vi "MultiPotentialStep.vi"() -> ()   [LabVIEW 2023]
uses:
  Sub_Vi/TypeDefs/Display.ctl
  Sub_Vi/TypeDefs/ChangeOnFly.ctl
  Sub_Vi/TypeDefs/Settings.ctl
  Sub_Vi/TypeDefs/WayPointCluster.ctl
  Settings.vi
panel:
  in  "t4 (s)":dbl
  in  "t3 (s)":dbl
  in  "t2 (s)":dbl
  in  "t1 (s)":dbl
  in  "E4 (V)":dbl
  in  "E2 (V)":dbl
  in  "E3 (V)":dbl
  in  "E1 (V)":dbl
  in  "SaveData?":bool=TRUE
  in  "WayPointCluster":T1
  in  "SettingsCluster":T2={"Sample Rate (us)"=1, "Samples Per Data Point (int, power of 2)"=1000, "DistanceToBulk (um)"=-1.0, "HoldTimeScaler"=1, "SaveData"=TRUE, "DistanceToBulk (um) 2"=-1.0, "DistanceToBulk (um) 3"=-1.0}
  in  "ChangeonFly":T3
  in  "Display Cluster":T4
  in  "stop":bool
  in  "Tab Control":enum32{"Current Followers", "Piezos"}(tab)
  out "E-t":dbl[](graph)
  out "i-t":dbl[](graph)
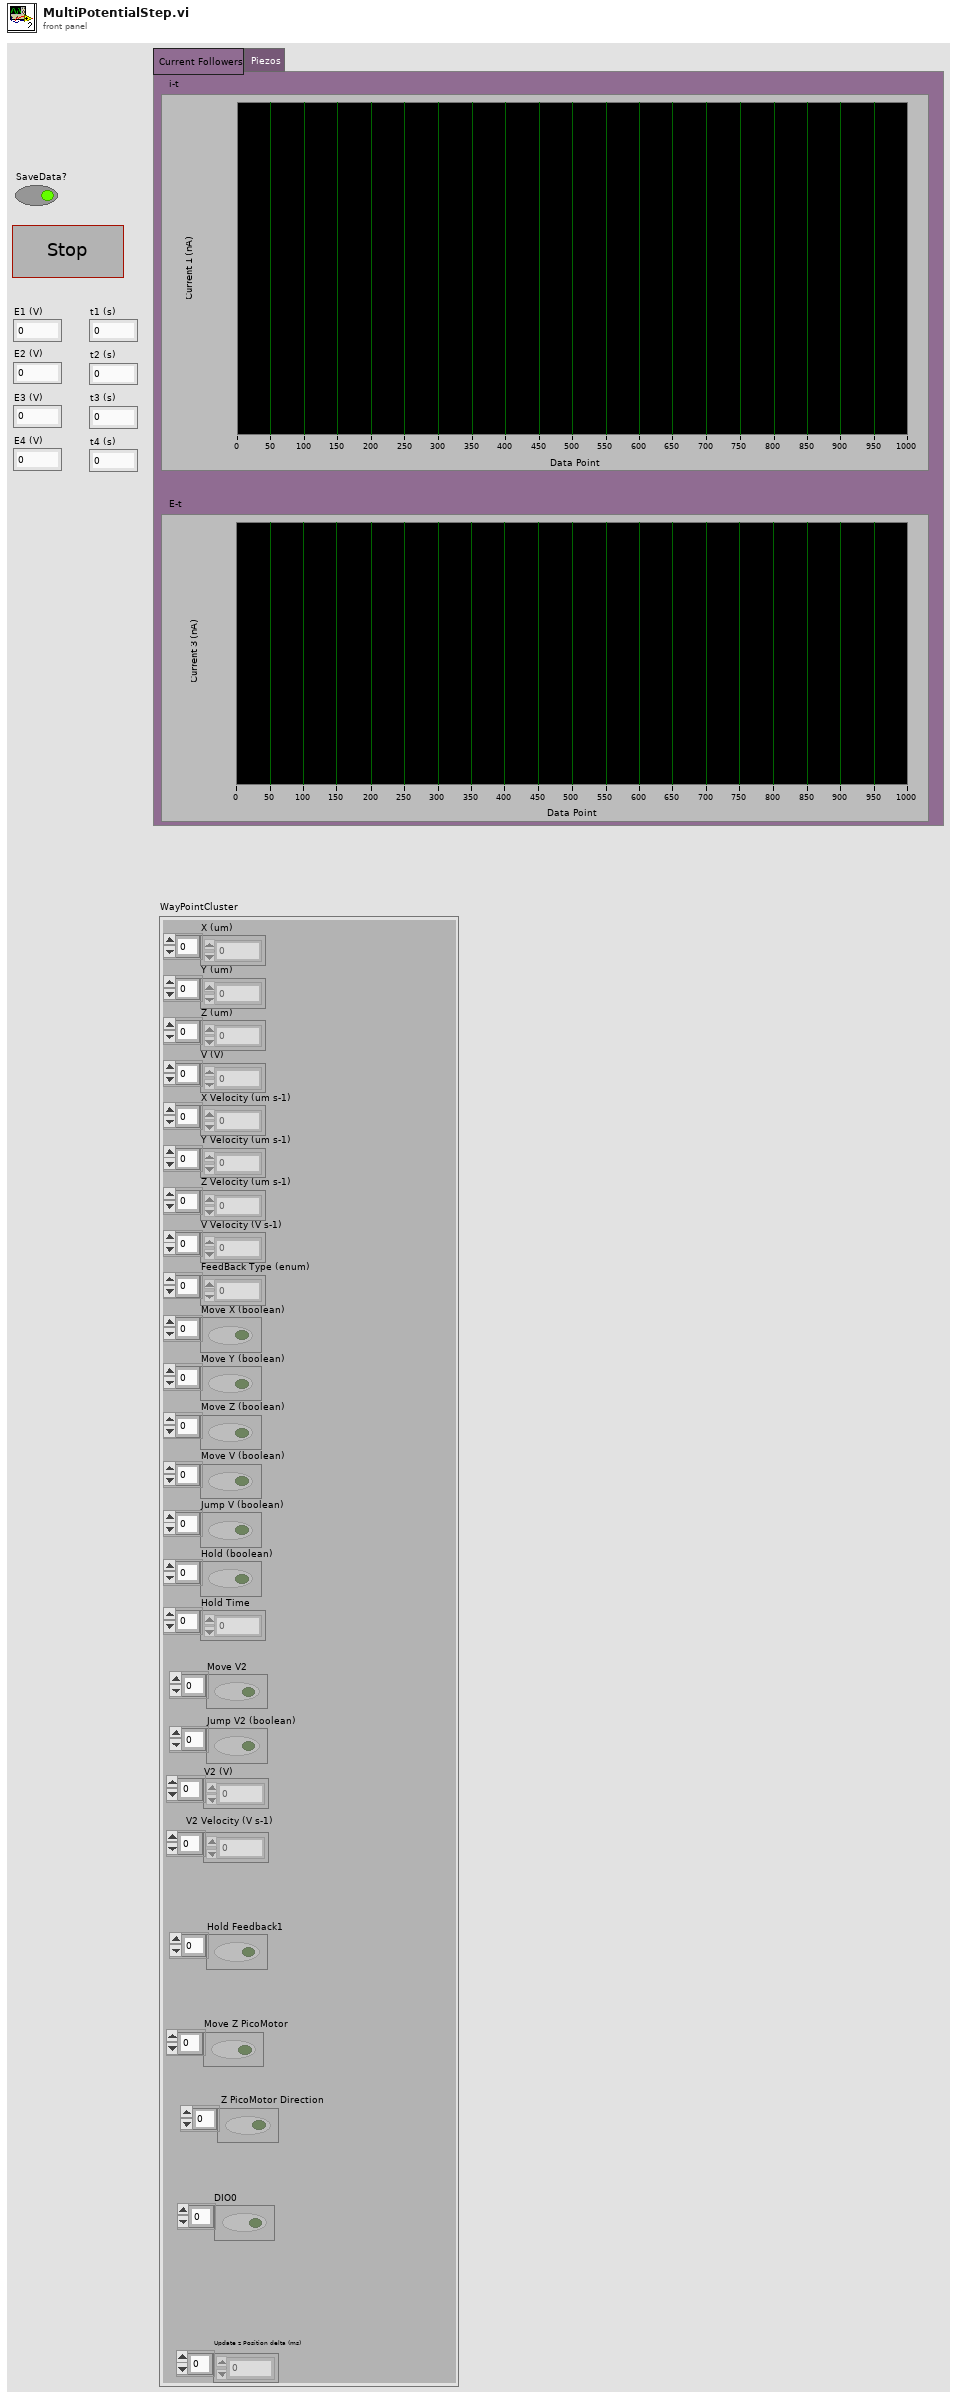
[diagram p1: front panel]
types:
  T1 = typedef "WayPointCluster.ctl" = cluster{"X (um)":dbl[], "Y (um)":dbl[], "Z (um)":dbl[], "V (V)":dbl[], "X Velocity (um s-1)":dbl[], "Y Velocity (um s-1)":dbl[], "Z Velocity (um s-1)":dbl[], "V Velocity (V s-1)":dbl[], "FeedBack Type (enum)":u16[], "Move X (boolean)":bool[], "Move Y (boolean)":bool[], "Move Z (boolean)":bool[], "Move V (boolean)":bool[], "Jump V (boolean)":bool[], "Hold (boolean)":bool[], "Hold Time":u32[], "V2 (V)":dbl[], "Move V2":bool[], "V2 Velocity (V s-1)":dbl[], "Jump V2 (boolean)":bool[], "Update z Position delta (ms)":i16[], "Hold Feedback1":bool[], "Move Z PicoMotor":bool[], " Z PicoMotor Direction":bool[], "DIO0":bool[]}
  T2 = typedef "Settings.ctl" = cluster{"Sample Rate (us)":u32, "Samples Per Data Point (int, power of 2)":i16, "DistanceToBulk (um)":dbl, "HoldTimeScaler":u64, "SaveData":bool, "DistanceToBulk (um) 2":dbl, "DistanceToBulk (um) 3":dbl}
  T3 = typedef "ChangeOnFly.ctl" = cluster{"Stop (boolean)":refnum<vi>, "Pause (boolean)":refnum<vi>, "EndCurrentLine (boolean)":refnum<vi>, "max movement per update step (Interger, nm)":refnum<vi>, "P (float, arb)":refnum<vi>, "Feedback set point (double, Amps)":refnum<vi>, "Voltage (double, V)":refnum<vi>, "Feedback set point 2 (double, Amps)":refnum<vi>, "Stop on Greater Than 2? (boolean)":refnum<vi>, "Stop on Greater Than? (boolean)":refnum<vi>, "Voltage 2 (double, V)":refnum<vi>, "Feedback Type (enum)":refnum<vi>, "Feedback Type 2 (enum)":refnum<vi>}
  T4 = typedef "Display.ctl" = cluster{"X":refnum<vi>, "Y":refnum<vi>, "Z":refnum<vi>, "Amp":refnum<vi>, "Phase":refnum<vi>, "t vs Z":refnum<vi>, "t vs C1":refnum<vi>, "t vs C2":refnum<vi>, "t vs C3":refnum<vi>, "t vs Amp":refnum<vi>, "t vs Phase":refnum<vi>, "t vs X":refnum<vi>, "t vs Y":refnum<vi>, "Z vs C1":refnum<vi>, "Z vs C2":refnum<vi>, "Z vs C3":refnum<vi>, "V vs C1":refnum<vi>, "V vs C2":refnum<vi>, "V vs C3":refnum<vi>, "X/Y/Z F":refnum<vi>, "X/Y/Z R":refnum<vi>, "X/Y/C1 F":refnum<vi>, "X/Y/C1 R":refnum<vi>, "X/Y/C2 F":refnum<vi>, "X/Y/C2 R":refnum<vi>, "X/Y/C3 F":refnum<vi>, "X/Y/C3 R":refnum<vi>, "NumberOfLines":u16, "um Per Pixel":dbl, "um Per Line":dbl, "X Center":dbl, "Hop X/Y/Z":refnum<vi>, "Hop X/Y/C1":refnum<vi>, "Hop X/Y/C2":refnum<vi>, "Hop X/Y/C3":refnum<vi>, "X Width":dbl, "Y Width":dbl, "Hopping Distance":dbl, "V2 vs C1":refnum<vi>, "V vs Phase":refnum<vi>, "Y Center":dbl, "Number of Pixels":dbl, "V2 vs C2":refnum<vi>, "V2 vs C3":refnum<vi>, "V vs y":refnum<vi>, "V2 vs y":refnum<vi>, "Z vs Amp":refnum<vi>, "Z vs Phase":refnum<vi>}
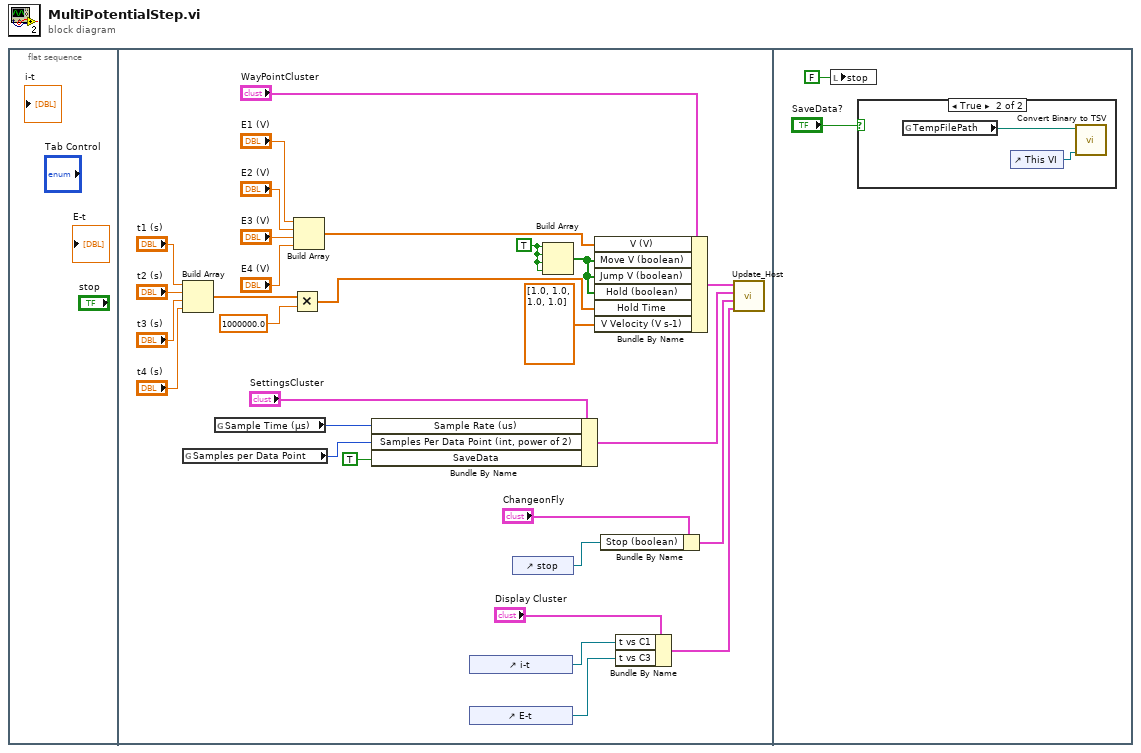
[diagram p0: block diagram]
diagram:
  n1 = flat-sequence {
    frame #0 {
    }
    frame #1 {
      w9 = TRUE ("Change V on Fly")
      n2 = Build Array("t1 (s)", "t2 (s)", "t3 (s)", "t4 (s)") -> (w2:dbl[])
      n3 = global read "Settings.vi" "Samples per Data Point"() -> (w24:u16)
      n4 = global read "Settings.vi" "Sample Time (µs)"() -> (w23:u32)
      n5 = Multiply(x=w2, y=1000000.0) -> (x*y=w4:dbl[])
      n6 = Build Array("E1 (V)", "E2 (V)", "E3 (V)", "E4 (V)") -> (w15:dbl[])
      n7 = Bundle By Name(cluster="SettingsCluster", "Sample Rate (us)"=w23, "Samples Per Data Point (int, power of 2)"=w24, "SaveData"=TRUE) -> (w21:T2)
      n8 = control-ref of="i-t"() -> (w18:refnum<vi>)
      n9 = control-ref of="E-t"() -> (w29:refnum<vi>)
      n10 = control-ref of="stop"() -> (w17:refnum<vi>)
      n11 = Build Array(w9, w9, w9, w9) -> (w10:bool[])
      n12 = Bundle By Name(cluster="WayPointCluster", "V (V)"=w15, "Move V (boolean)"=w10, "Jump V (boolean)"=w10, "Hold (boolean)"=w10, "Hold Time"=w4, "V Velocity (V s-1)"=dbl[] [1.0, 1.0, 1.0, 1.0]) -> (w22:T1)
      n13 = Bundle By Name(cluster="ChangeonFly", "Stop (boolean)"=w17) -> (w19:T3)
      n14 = Bundle By Name(cluster="Display Cluster", "t vs C1"=w18, "t vs C3"=w29) -> (w20:T4)
      n15 = call "Update_Host.vi"("Display Cluster"=w20, "ChangeonFly"=w19, "SettingsCluster"=w21, "WayPointCluster"=w22) -> ()  [unwired: 6 in]
    }
    frame #2 {
      n16 = local write "stop"(FALSE ("stop")) -> ()
      n17 = case shown="True" "SaveData?" {
        frame False {
        }
        frame True {
          n18 = global read "Settings.vi" "TempFilePath"() -> (w32:path)
          n19 = control-ref of="This VI"() -> (w33:refnum<vi>)
          n20 = call "Convert Binary to TSV.vi"("This VI"=w33, "TDMS DataFile Name"=w32) -> ()  [unwired: 10 in]
        }
      }
    }
  }
